vi "create_task.vi"(8 "error in (no error)":errorcluster, 11 "SignalWriterDL101123SoundCard in":refnum<class "SignalWriterDL101123SoundCard.lvclass">) -> (0 "error out":errorcluster, 3 "SignalWriterDL101123SoundCard out":refnum<class "SignalWriterDL101123SoundCard.lvclass">)   [LabVIEW 2010, in "SignalWriterDL101123SoundCard.lvclass"]
uses:
  SignalWriterDL101123SoundCard.lvclass
  <vilib>/sound2/lvsound2.llb/Sound Data Format.ctl
  <vilib>/sound2/lvsound2.llb/Sampling Mode.ctl
  SignalWriterDL101123SoundCard.lvclass/SignalWriterDL101123SoundCard.ctl
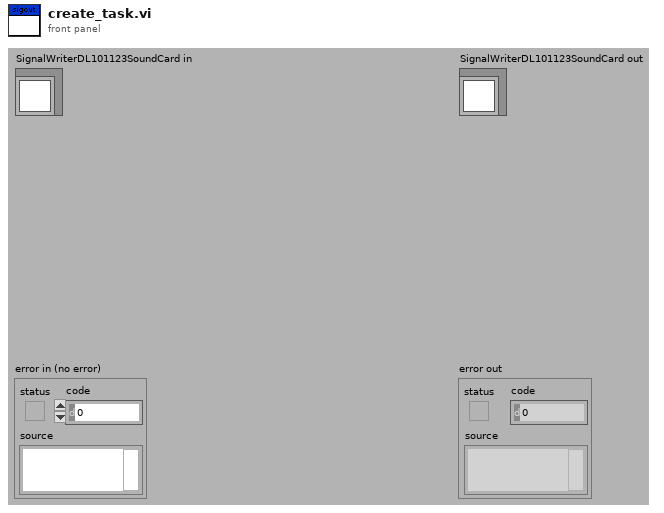
[diagram p1: front panel]
types:
  T1 = typedef "Sound Data Format.ctl" = cluster{"sample rate (S/s)":dbl, "number of channels":i32, "bits per sample":i32}
  T2 = typedef "Sampling Mode.ctl" = i32
  T3 = typedef "Sound Output Task ID.ctl" = u32
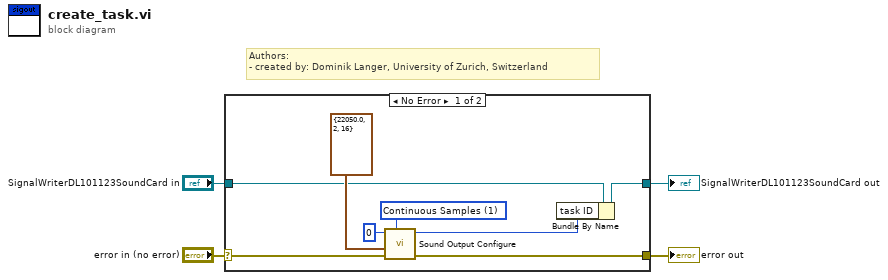
[diagram p0: block diagram]
diagram:
  # "Authors: \n- created by: Dominik Langer, University of Zurich, Switzerland"
  n1 = case shown="No Error" "error in (no error)" {
    selector: "error in (no error)" -> [w12 w14]
    tunnel: [w11 w14] -> w3
    tunnel: [w5 w13] -> w1
    tunnel: "SignalWriterDL101123SoundCard in" -> [w6 w13]
    frame No Error {
      w10 = T2 1 items=["Finite Samples", "Continuous Samples"] ("sample mode")
      n2 = call <vilib>:"Sound Output Configure.vi"("sample mode"=w10, "error in (no error)"=w12, "sound format"=T1 {"sample rate (S/s)"=22050.0, "number of channels"=2, "bits per sample"=16}, "device ID"=u32 0) -> ("error out"=w11:errorcluster, "task ID"=w7:T3)  [unwired: 6 in]
      n3 = Bundle By Name(cluster=w6, "task ID"=w7) -> (w5:refnum<class "SignalWriterDL101123SoundCard.lvclass">)
    }
    frame Error {
    }
  }
  "error out" <- w3
  "SignalWriterDL101123SoundCard out" <- w1
